vi "Fetch Multi Eval Meas List ACLR NR Carrier Frequency Results.vi"(7 "Carrier Frequency (Negative)":i32(ring) items=["Negative", "Positive"], 8 "error in (no error)":errorcluster, 9 "Result Type (Current)":i32(ring) items=["Current", "Average"], 10 "Instance (1)":T1=1, 11 "VISA resource name":refnum<visa-resource-name>) -> (0 "error out":errorcluster, 1 "ACLR NR Carrier Frequency Results":dbl[](array[numeric]) format="%#.9p", 2 "Reliability":i32, 3 "VISA resource name out":refnum<visa-resource-name>)   [LabVIEW 2015, in "Rohde&Schwarz CMXP NR FR2 Measurement.lvlib"]
doc: "Returns the power in the allocated NR channel for all measured list mode segments.\n\nAttributes:\nRSCMXPNRFR2M_ATTR_FETCH_MULTI_EVAL_MEASUREMENT_LIST_ACLR_NR_NEGATIVE_AVERAGE_RESULTS\nRSCMXPNRFR2M_ATTR_FETCH_MULTI_EVAL_MEASUREMENT_LIST_ACLR_NR_NEGATIVE_CURRENT_RESULTS\nRSCMXPNRFR2M_ATTR_FETCH_MULTI_EVAL_MEASUREMENT_LIST_ACLR_NR_POSITIVE_AVERAGE_RESULTS\nRSCMXPNRFR2M_ATTR_FETCH_MULTI_EVAL_MEASUREMENT_LIST_ACLR_NR_POSITIVE_CURRENT_RESULTS\n\nRemote-control commands:\nFETCh:NRMMw:MEAS<i>:MEValuation:LIST:ACLR:NR:NEGativ:AVERage?\nFETCh:NRMMw:MEAS<i>:MEValuation:LIST:ACLR:NR:NEGativ:CURRent?\nFETCh:NRMMw:MEAS<i>:MEValuation:LIST:ACLR:NR:POSitiv:AVERage?\nFETCh:NRMMw:MEAS<i>:MEValuation:LIST:ACLR:NR:POSitiv:CURRent?"
uses:
  <instrlib>/Rohde&Schwarz CMXP NR FR2 Measurement/Rohde&Schwarz CMXP NR FR2 Measurement.lvlib
  <instrlib>/Rohde&Schwarz CMXP NR FR2 Measurement/Private/_Instance.ctl
  <instrlib>/Rohde&Schwarz CMXP NR FR2 Measurement/Private/rsidr_core.llb/rsidr_core.lvlib
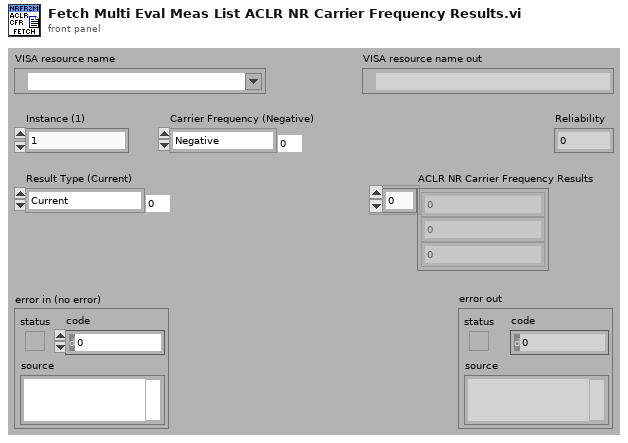
[diagram p1: front panel]
types:
  T1 = typedef "Rohde&Schwarz CMXP NR FR2 Measurement.lvlib/_Instance.ctl" = i32
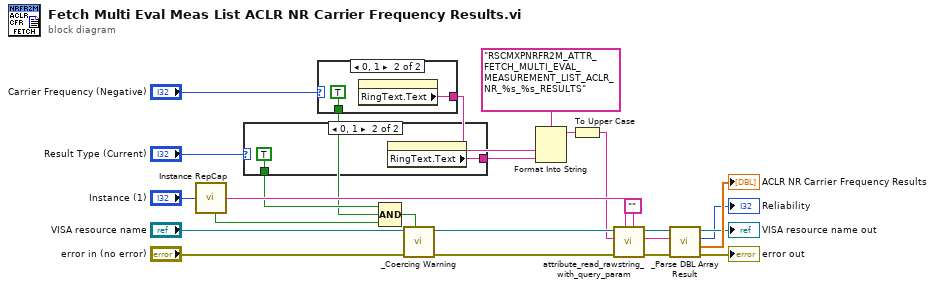
[diagram p0: block diagram]
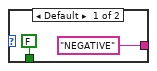
[diagram p2: hidden frame]
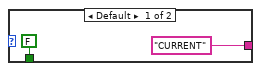
[diagram p3: hidden frame]
diagram:
  n1 = call <instrlib>:"Instance RepCap.vi"("Instance In"="Instance (1)") -> ("In Range?"=w18:bool, "RepCap Identifier Out"=w22:string)  [unwired: 1 in]
  n2 = case shown="0, 1" "Result Type (Current)" {
    tunnel: ["CURRENT" w28] -> w19
    tunnel: [FALSE TRUE] -> w3
    frame Default {
    }
    frame 0, 1 {
      n3 = property on="Result Type (Current)" class="Ring (strict)"() -> ("RingText.Text"=w28:string)  [unwired: 2 in, 2 out]
    }
  }
  n4 = case shown="0, 1" "Carrier Frequency (Negative)" {
    tunnel: ["NEGATIVE" w32] -> w4
    tunnel: [FALSE TRUE] -> w1
    frame Default {
    }
    frame 0, 1 {
      n5 = property on="Carrier Frequency (Negative)" class="Ring (strict)"() -> ("RingText.Text"=w32:string)  [unwired: 2 in, 2 out]
    }
  }
  n6 = Compound Arithmetic op=AND(w3, w1, w18) -> (w17:bool)
  n7 = call <instrlib>:"_Coercing Warning.vi"("In Range?"=w17, "error in (no error)"="error in (no error)", "VISA resource name"="VISA resource name") -> ("error out"=w24:errorcluster, "VISA resource name out"=w23:refnum<visa-resource-name>)  [unwired: 7 in]
  n8 = Format Into String(format string="RSCMXPNRFR2M_ATTR_FETCH_MULTI_EVAL_MEASUREMENT_LIST_ACLR_NR_%s_%s_RESULTS", w4, w19) -> (resulting string=w21:string)  [unwired: 2 in, 1 out]
  n9 = To Upper Case(1:w21) -> (0:w20:string)
  n10 = call <instrlib>:"attribute_read_rawstring_with_query_param.vi"("Query Parameter (None)"="" ("Empty String Constant"), "Repeated Capability"=w22, "error in"=w24, "Attribute ID"=w20, "VISA resource name"=w23) -> ("error out"=w11:errorcluster, "Raw String out"=w10:string, "VISA resource name out"=w9:refnum<visa-resource-name>)  [unwired: 4 in]
  n11 = call <instrlib>:"_Parse DBL Array Result.vi"("error in (no error)"=w11, "Input String"=w10, "VISA resource name"=w9) -> ("error out"=→"error out":errorcluster, "Results"=→"ACLR NR Carrier Frequency Results":dbl[], "Reliability"=→"Reliability":i32, "VISA resource name out"=→"VISA resource name out":refnum<visa-resource-name>)  [unwired: 5 in]
